vi "CMD_Switch.vi"(1 "Line":string) -> (0 "Done":bool)   [LabVIEW 2013]
uses:
  <vilib>/Rock Robotics/WPI/Solenoid/WPI_SolenoidValue.ctl
  <vilib>/Rock Robotics/WPI/Solenoid/WPI_SolenoidSetEnum.vi
panel:
  in  "Parameters":i32[](array[numeric])=[1, 1, 1, 1]
  in  "Subcommands":string[](array[string])=["forward", "reverse", "on", "off"]
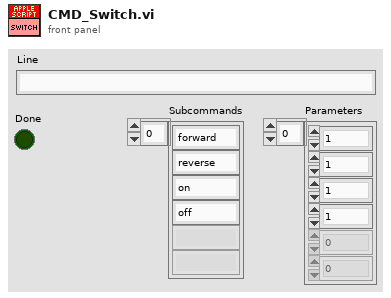
[diagram p1: front panel]
types:
  T1 = typedef "WPI_SolenoidValue.ctl" = enum16{"Off", "On", "Forward", "Reverse"}
  T2 = typedef "WPI_SolenoidDevRef.ctl" = cluster{"DevStatus":errorcluster, "Solenoid Module":T3, "Forward Solenoid Channel":T4, "Reverse Solenoid Channel":T4}
  T3 = typedef "FPGA_TypedefSolenoidModule.ctl" = enum16{"Solenoid Module 1", "Solenoid Module 2"}
  T4 = typedef "WPI_SolenoidChannel.ctl" = enum8{"Solenoid 1", "Solenoid 2", "Solenoid 3", "Solenoid 4", "Solenoid 5", "Solenoid 6", "Solenoid 7", "Solenoid 8", "Invalid"}
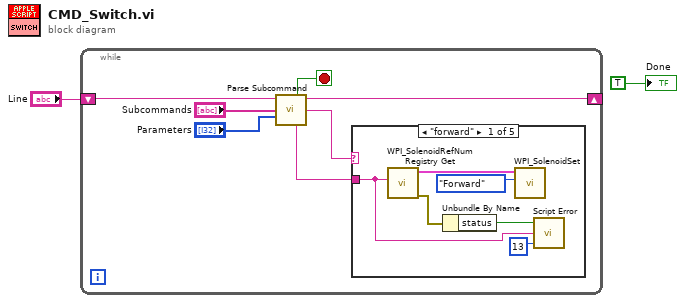
[diagram p0: block diagram]
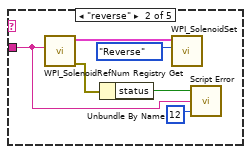
[diagram p2: hidden frame]
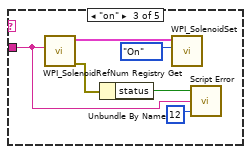
[diagram p3: hidden frame]
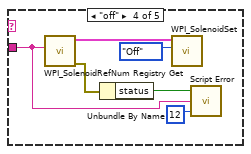
[diagram p4: hidden frame]
diagram:
  n1 = while {
    shift-right: [w6] -> _
    shift-left: "Line" -> [w9]
    stop <- w5 stop-if-true
    n2 = call "Parse Subcommand.vi"("Text In"=w9, "Subcommands"="Subcommands", "Parameters"="Parameters") -> ("Done"=w5:bool, "Text Out"=w6:string, "Subcommand"=w4:string, "Parameter 1"=w3:string)  [unwired: 6 in, 3 out]
    n3 = case shown="\"forward\"" w4 {
      tunnel: w3 -> [w11 w17 w23 w29 _]
      frame "forward" {
        n4 = call <vilib>:"WPI_SolenoidRefNum Registry Get.vi"("refnum name"=w11) -> ("error out"=w13:errorcluster, "SolenoidDevRef"=w15:T2)  [unwired: 9 in]
        n5 = Unbundle By Name(w13) -> ("status"=w12:bool)
        n6 = call-poly <vilib>:"WPI_SolenoidSet.vi"("Value"=WPI_SolenoidValue."Forward", "SolenoidDevRef"=w15) -> ()  [unwired: 8 in, 2 out]
        n7 = call "Script Error.vi"("Error?"=w12, "Error Details"=w11, "Error Code"=13) -> ()  [unwired: 3 in]
      }
      frame "reverse" {
        n8 = call <vilib>:"WPI_SolenoidRefNum Registry Get.vi"("refnum name"=w17) -> ("error out"=w19:errorcluster, "SolenoidDevRef"=w21:T2)  [unwired: 9 in]
        n9 = Unbundle By Name(w19) -> ("status"=w18:bool)
        n10 = call-poly <vilib>:"WPI_SolenoidSet.vi"("Value"=WPI_SolenoidValue."Reverse", "SolenoidDevRef"=w21) -> ()  [unwired: 8 in, 2 out]
        n11 = call "Script Error.vi"("Error?"=w18, "Error Details"=w17, "Error Code"=12) -> ()  [unwired: 3 in]
      }
      frame "on" {
        n12 = call <vilib>:"WPI_SolenoidRefNum Registry Get.vi"("refnum name"=w23) -> ("error out"=w25:errorcluster, "SolenoidDevRef"=w27:T2)  [unwired: 9 in]
        n13 = Unbundle By Name(w25) -> ("status"=w24:bool)
        n14 = call-poly <vilib>:"WPI_SolenoidSet.vi"("Value"=WPI_SolenoidValue."On", "SolenoidDevRef"=w27) -> ()  [unwired: 8 in, 2 out]
        n15 = call "Script Error.vi"("Error?"=w24, "Error Details"=w23, "Error Code"=12) -> ()  [unwired: 3 in]
      }
      frame "off" {
        n16 = call <vilib>:"WPI_SolenoidRefNum Registry Get.vi"("refnum name"=w29) -> ("error out"=w31:errorcluster, "SolenoidDevRef"=w33:T2)  [unwired: 9 in]
        n17 = Unbundle By Name(w31) -> ("status"=w30:bool)
        n18 = call-poly <vilib>:"WPI_SolenoidSet.vi"("Value"=WPI_SolenoidValue."Off", "SolenoidDevRef"=w33) -> ()  [unwired: 8 in, 2 out]
        n19 = call "Script Error.vi"("Error?"=w30, "Error Details"=w29, "Error Code"=12) -> ()  [unwired: 3 in]
      }
      frame Default {
      }
    }
  }
  "Done" <- TRUE
